vi "read log file.vi"(11 "file (use dialog)":path) -> (3 "array":string[](array[string]))   [LabVIEW 2023]
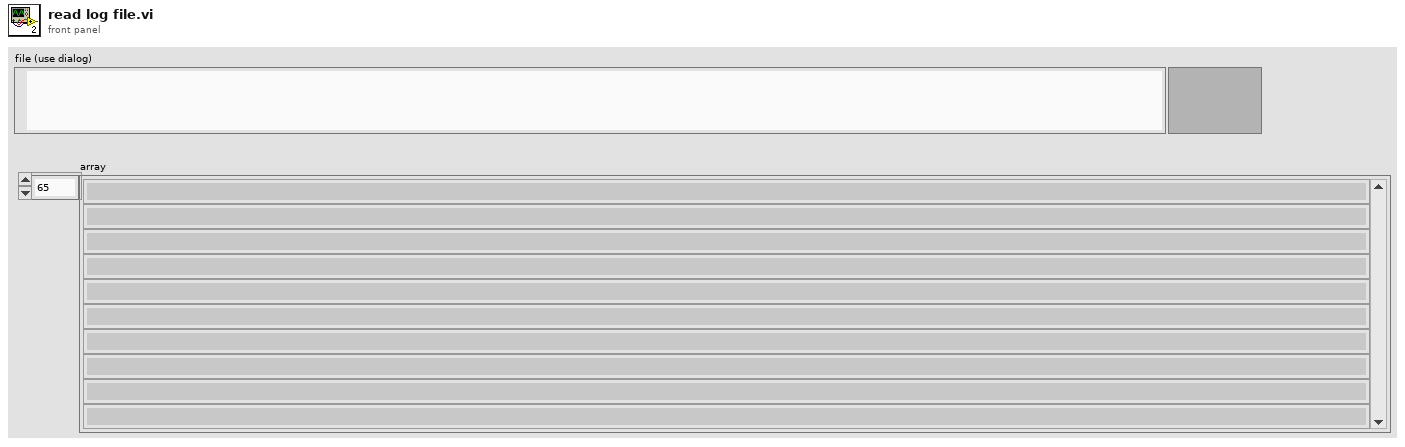
[diagram p1: front panel]
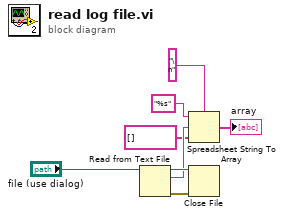
[diagram p0: block diagram]
diagram:
  n1 = Read from Text File(file (use dialog)="file (use dialog)") -> (refnum out=w6:refnum<file>, text=w5:string, error out=w7:errorcluster)  [unwired: 3 in, 1 out]
  n2 = Spreadsheet String To Array(delimiter (Tab)="\n", format string="%s", spreadsheet string=w5, array type (2D Dbl)=string[] []) -> (array=→"array":string[])
  n3 = Close File(refnum=w6, error in=w7) -> ()  [unwired: 2 out]
